vi "Rename Slave Node.vi"(7 "Prepend":bool, 8 "error in (no error)":errorcluster, 9 "Slave #":u16, 10 "Slave Name":string, 11 "Item Ref in":T1 format="%.0x") -> (0 "error out":errorcluster, 3 "Item Ref out":T1 format="%.0x")   [LabVIEW 2020, in "SEECD System Explorer.lvlib"]
uses:
  SEECD System Explorer.lvlib
  <vilib>/NI VeriStand/Custom Device API/Custom Device API.lvlib
  <vilib>/NI VeriStand/Custom Device API/Custom Device Item Ref.ctl
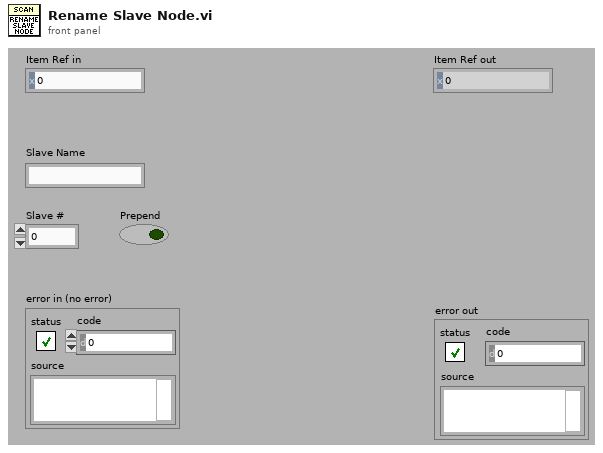
[diagram p1: front panel]
types:
  T1 = typedef "Custom Device API.lvlib/Custom Device Item Ref.ctl" = u64
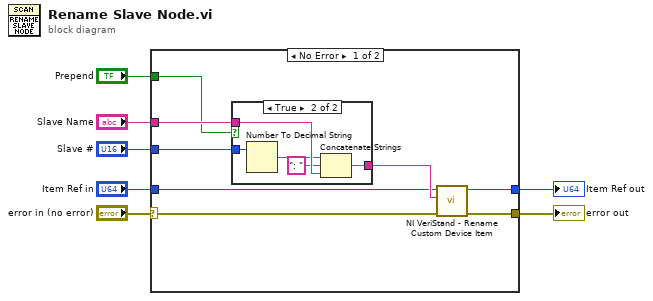
[diagram p0: block diagram]
diagram:
  n1 = case shown="No Error" "error in (no error)" {
    selector: "error in (no error)" -> [w9 w22]
    tunnel: "Item Ref in" -> [w8 w23]
    tunnel: "Slave Name" -> [w14 _]
    tunnel: "Slave #" -> [w13 _]
    tunnel: [w10 w22] -> w3
    tunnel: [w11 w23] -> w2
    tunnel: "Prepend" -> [w12 _]
    frame No Error {
      n2 = case shown="True" w12 {
        tunnel: [w16 w21] -> w15
        tunnel: w14 -> [w16 w20]
        tunnel: w13 -> [_ w19]
        frame False {
        }
        frame True {
          n3 = Number To Decimal String(number=w19) -> (decimal integer string=w18:string)  [unwired: 1 in]
          n4 = Concatenate Strings(w18, ": " ("string"), w20) -> (w21:string)
        }
      }
      n5 = call <vilib>:"NI VeriStand - Rename Custom Device Item.vi"("error in (no error)"=w9, "New Name"=w15, "Item Ref in"=w8) -> ("error out"=w10:errorcluster, "Item Ref out"=w11:T1)  [unwired: 1 in, 6 out]
    }
    frame Error {
    }
  }
  "error out" <- w3
  "Item Ref out" <- w2
